vi "CenterHolo.vi"(8 "X":dbl, 9 "Y":dbl, 11 "Holo Size":i32) -> (0 "X centered":i32, 1 "Y centered":i32)   [LabVIEW 2018]
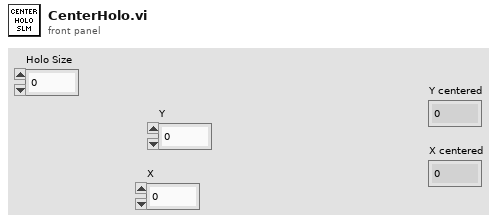
[diagram p1: front panel]
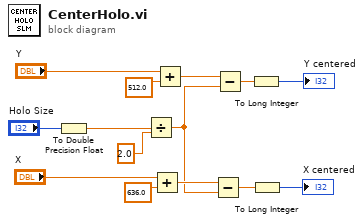
[diagram p0: block diagram]
diagram:
  n1 = To Double Precision Float(number="Holo Size") -> (double precision float=w3:dbl)
  n2 = Divide(x=w3, y=2.0) -> (x/y=w11:dbl)
  n3 = Add(x="X", y=636.0 ("x")) -> (x+y=w13:dbl)
  n4 = Add(x="Y", y=512.0 ("x")) -> (x+y=w12:dbl)
  n5 = Subtract(x=w13, y=w11) -> (x-y=w8:dbl)
  n6 = Subtract(x=w12, y=w11) -> (x-y=w7:dbl)
  n7 = To Long Integer(number=w7) -> (32bit integer=→"Y centered":i32)
  n8 = To Long Integer(number=w8) -> (32bit integer=→"X centered":i32)
